vi "DeInit.vi"(8 "error in (no error)":errorcluster, 11 "Master in":refnum<class "Master.lvclass">) -> (0 "error out":errorcluster, 3 "Master out":refnum<class "Master.lvclass">)   [LabVIEW 2021, in "Master.lvlib" / "Master.lvclass"]
uses:
  Master.lvclass
  Slave/Clone Registration/Clone Registration.lvlib
  Slave/Slave.lvlib
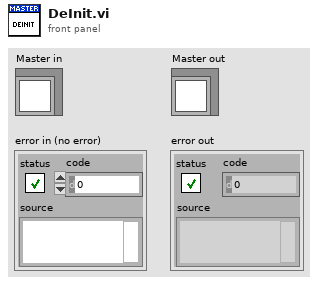
[diagram p1: front panel]
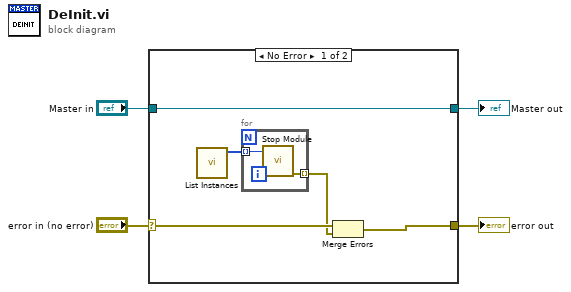
[diagram p0: block diagram]
diagram:
  n1 = case shown="No Error" "error in (no error)" {
    selector: "error in (no error)" -> [w8 w13]
    tunnel: [w6 w13] -> w3
    tunnel: [w9 w12] -> w1
    tunnel: "Master in" -> [w9 w12]
    frame No Error {
      n2 = call "List Instances.vi"() -> ("Module IDs"=w7:i32[])  [unwired: 7 in, 4 out]
      n3 = for {
        tunnel: w7 -> [w11] mode=indexing
        tunnel: [w10] -> w5 mode=indexing
        n4 = call "Stop Module.vi"("Module ID"=w11) -> ("error out"=w10:errorcluster)  [unwired: 10 in]
      }
      n5 = Merge Errors(w8, w5) -> (w6:errorcluster)
    }
    frame Error {
    }
  }
  "error out" <- w3
  "Master out" <- w1
